vi "FRCts20_Backend_Event_PPD_return.vi"(7 "Event":T1, 8 "error in (no error)":errorcluster, 9 "rows affected 2":i32, 10 "rows affected":i32) -> (0 "error out":errorcluster, 3 "data string":string)   [LabVIEW 2014, in "FRCts20_Backend_Engine.lvlib"]
doc: "Returns whether an event was successfully updated or deleted"
uses:
  FRCts20_Backend_Engine.lvlib
  FRCts20_Backend_API/FRCts20_Backend_API_Event.ctl
  FRCts20_Backend_API/FRCts20_Backend_API_SW.ctl
  FRCts20_Backend_API/FRCts20_Backend_API.lvlib
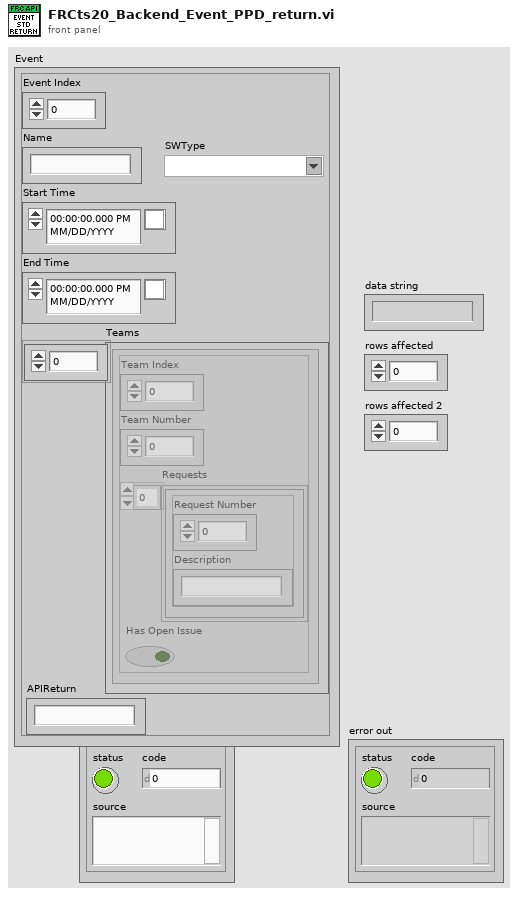
[diagram p1: front panel]
types:
  T1 = typedef "FRCts20_Backend_API.lvlib/FRCts20_Backend_API_Event.ctl" = cluster{"Event Index":u32, "Name":string, "Start Time":timestamp, "End Time":timestamp, "Teams":cluster{"Team Index":u32, "Team Number":u32, "Requests":cluster{"Request Number":u32, "Description":string}[], "Has Open Issue":bool}[], "SWType":T2, "APIReturn":string}
  T2 = typedef "FRCts20_Backend_API.lvlib/FRCts20_Backend_API_SW.ctl" = string
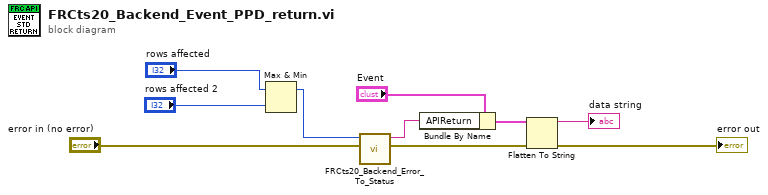
[diagram p0: block diagram]
diagram:
  n1 = Max & Min(x="rows affected", y="rows affected 2") -> (max(x,y)=w1:i32)  [unwired: 1 out]
  n2 = call "FRCts20_Backend_Error_To_Status.vi"("error in (no error)"="error in (no error)", "rows affected"=w1) -> ("error out"=w7:errorcluster, "String"=w8:string)  [unwired: 8 in]
  n3 = Bundle By Name(cluster="Event", "APIReturn"=w8) -> (w6:T1)
  n4 = Flatten To String(anything=w6, error in (no error)=w7) -> (data string=→"data string":string, error out=→"error out":errorcluster)  [unwired: 2 in, 1 out]
